vi "Knock Sensor 1.0 In Place Input Write Structure.vi"(5 "Device Inputs":dbl[](array[numeric]), 7 "Last Device Inputs":dbl[](array[numeric]), 8 "error in (no error)":errorcluster, 9 "FPGA ref in":T1, 11 "1.0.0 Knock Sensor in":T2) -> (0 "error out":errorcluster, 1 "FPGA ref out":T1, 3 "1.0.0 Knock Sensor out":T2)   [LabVIEW 2017, in "Engine Simulation Toolkit Engine.lvlib"]
uses:
  Engine Simulation Toolkit Engine.lvlib
  Shared/1.0 Knock Sensor Engine Data.ctl
  Shared/1.0 Knock Sensor FIFO Idxs.ctl
  Knock Sensor 1.0 Input Ref.ctl
  Knock Sensor 1.0 FPGA Inputs Write Node.vi
  Shared/Engine Simulation Toolkit Shared.lvlib
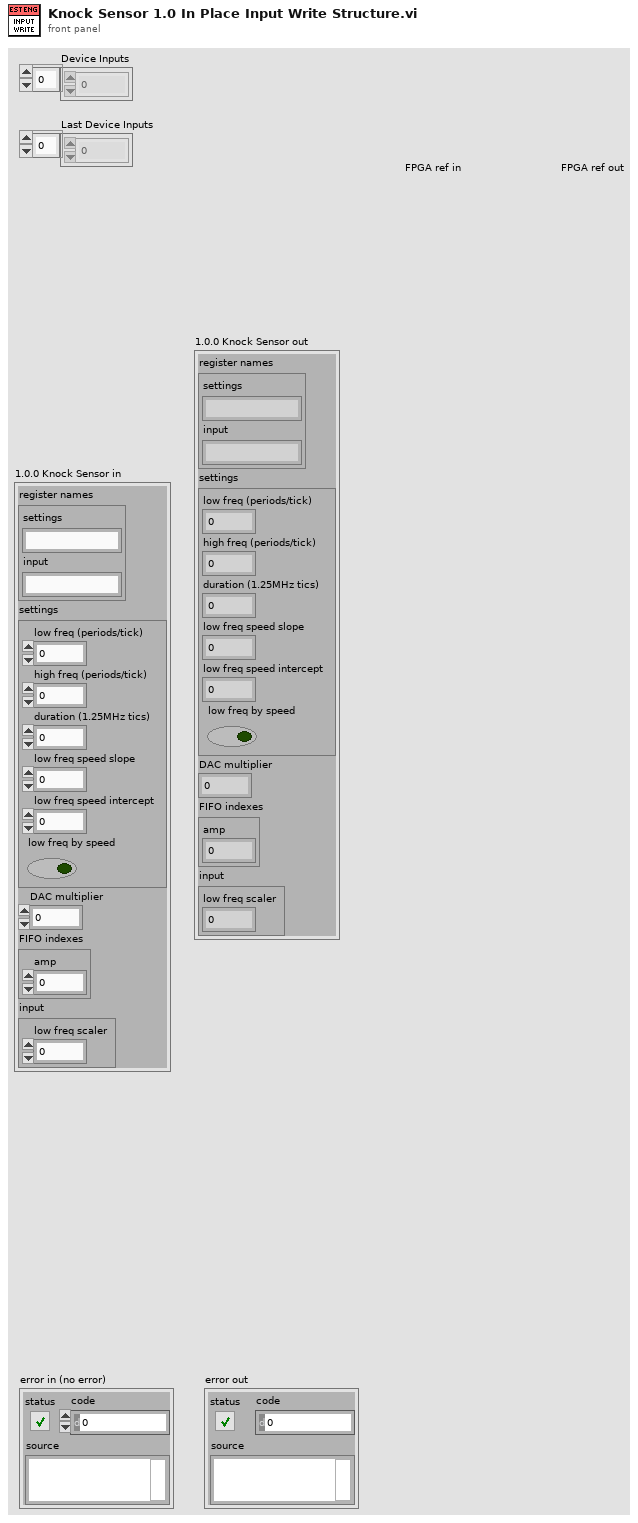
[diagram p1: front panel]
types:
  T1 = typedef "Engine Simulation Toolkit Engine.lvlib/Knock Sensor 1.0 Input Ref.ctl" = refnum<k20>
  T2 = typedef "Engine Simulation Toolkit Shared.lvlib/1.0 Knock Sensor Engine Data.ctl" = cluster{"register names":cluster{"settings":string, "input":string}, "settings":cluster{"low freq (periods/tick)":fxp<+,32,0>, "high freq (periods/tick)":fxp<+,32,0>, "duration (1.25MHz tics)":fxp<+,18,18>, "low freq speed slope":fxp<+,16,-3>, "low freq speed intercept":fxp<+,10,-10>, "low freq by speed":bool}, "DAC multiplier":dbl, "FIFO indexes":T3, "input":cluster{"low freq scaler":fxp<+,10,0>}}
  T3 = typedef "Engine Simulation Toolkit Shared.lvlib/1.0 Knock Sensor FIFO Idxs.ctl" = cluster{"amp":i32}
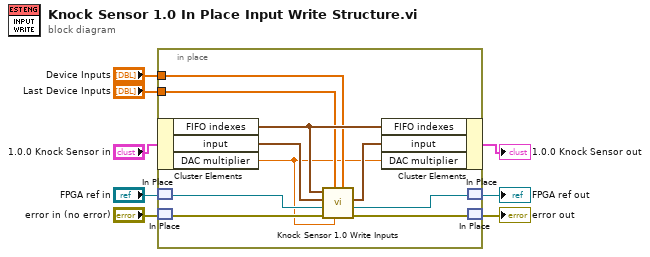
[diagram p0: block diagram]
diagram:
  n1 = in-place {
    in-place-border: "Last Device Inputs" -> [w13]
    in-place-border: "Device Inputs" -> [w12]
    n2 = in-place-cluster #1("1.0.0 Knock Sensor in") -> ("FIFO indexes"=w15:T3, "input"=w16:cluster{"low freq scaler":fxp<+,10,0>}, "DAC multiplier"=w9:dbl)
    n3 = in-place-match #2("FPGA ref in") -> (w11:T1)
    n4 = in-place-match #3("error in (no error)") -> (w18:errorcluster)
    n5 = call "Knock Sensor 1.0 Write Inputs.vi"("Device inputs"=w12, "DAC multiplier"=w9, "Last Device inputs"=w13, "error in (no error)"=w18, "input reference in"=w11, "input in"=w16, "FIFO indexes.inputs"=w15) -> ("error out"=w17:errorcluster, "input reference out"=w10:T1, "input out"=w14:cluster{"low freq scaler":fxp<+,10,0>})  [unwired: 2 in]
    n6 = in-place-cluster #1("FIFO indexes"=w15, "input"=w14, "DAC multiplier"=w9) -> (→"1.0.0 Knock Sensor out":T2)
    n7 = in-place-match #2(w10) -> (→"FPGA ref out":T1)
    n8 = in-place-match #3(w17) -> (→"error out":errorcluster)
  }
